vi "subFILEmain.vi"(6 "Trial":string, 9 "Test":string caption="Participant Name (FirstLast)", 10 "Folder name: Participant":string caption="Participant Name (FirstLast)", 11 "File Folder":path=path "C:/Users/rsKite/Desktop/FSR DATA") -> (0 "error out":errorcluster, 2 "File Name":string, 3 "refnum out":refnum<file>)   [LabVIEW 2020]
panel:
  in  "Hand":string caption="Participant Name (FirstLast)"
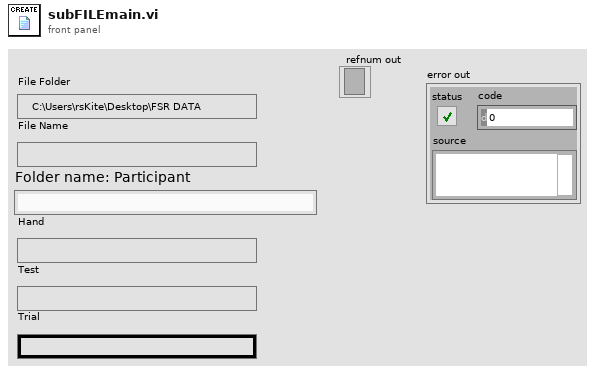
[diagram p1: front panel]
types:
  T1 = enum16{"open", "replace", "create", "open or create", "replace or create", "replace or create with confirmation"}
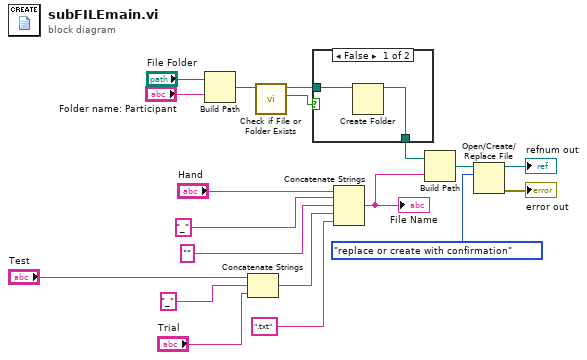
[diagram p0: block diagram]
diagram:
  n1 = Build Path(base path="File Folder", name or relative path="Folder name: Participant") -> (appended path=w15:path)
  n2 = Concatenate Strings("Test", "_" ("string"), "Trial") -> (w5:string)
  n3 = call <vilib>:"Check if File or Folder Exists.vi"("path"=w15) -> ("file or folder exists?"=w18:bool, "dup path"=w17:path)  [unwired: 8 in, 1 out]
  n4 = case shown="False" w18 {
    tunnel: w17 -> [w21 w22]
    tunnel: [w20 w22] -> w19
    frame False {
      n5 = Create Folder(path (use dialog)=w21) -> (created path=w20:path)  [unwired: 2 in, 2 out]
    }
    frame True {
    }
  }
  n6 = Concatenate Strings("Hand", "_" ("string"), "" ("string"), w5, ".txt" ("string")) -> (w12:string)
  "File Name" <- w12
  n7 = Build Path(base path=w19, name or relative path=w12) -> (appended path=w4:path)
  n8 = Open/Create/Replace File(file path (use dialog)=w4, operation (0:open)=T1."replace or create with confirmation") -> (refnum out=→"refnum out":refnum<file>, error out=→"error out":errorcluster)  [unwired: 4 in, 1 out]
